vi "cv_04-06.vi"() -> ()   [LabVIEW 2013]
panel:
  out "Array 2":u16[](array[numeric])
  out "Array":u16[](array[numeric])
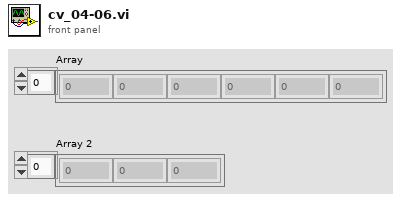
[diagram p1: front panel]
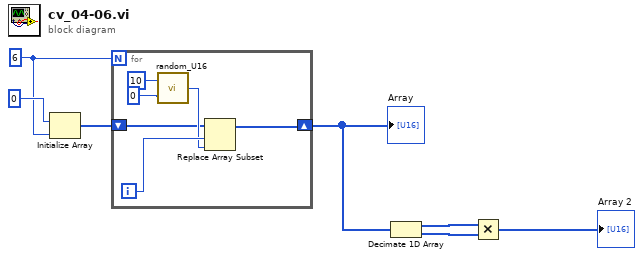
[diagram p0: block diagram]
diagram:
  w5 = 6
  n1 = Initialize Array(0, w5) -> (w6:i32[])
  n2 = for {
    N: w5 -> [_]
    shift-right: [w8] -> w4
    shift-left: w6 -> [w9]
    i -> [w13]
    n3 = call "random_U16.vi"("Offset"=0, "Range"=10) -> ("Out"=w12:u16)
    n4 = Replace Array Subset(array=w9, new element=w12, index=w13) -> (w8:i32[])
  }
  "Array" <- w4
  n5 = Decimate 1D Array(w4) -> (w3:i32[], w2:i32[])
  n6 = Multiply(x=w3, y=w2) -> (x*y=→"Array 2":i32[])
